vi "CreateNewWizard_Init.vi"(11 "Wizard":T1) -> (1 "Label":string, 2 "Enable Finish":bool, 3 "Enable Next":bool)   [LabVIEW 2020, in "Add Actor.lvlib"]
doc: "NI Confidential \n\n/**\n@brief This VI is called by the framework when an item of this type is first created.\n\n@author Joel Dixon\n\n@par Sample_Item_Init.vi\n This VI might typically set the popup menu for this item by calling mxLvSetPopupMenu.vi, set the icon for the item by calling mxLvSetIcon.vi, and set a name to be displayed in the tree by calling mxLvSetName.vi. \n\n@param \"Object\" [in] \nPassed by the framework as a reference to 'this' item in the tree. This parameter can be passed as the 'item' parameter for any of the mxLv** VIs, such as mxLvCreateItems.vi.\n*/"
uses:
  Add Actor.lvlib
  Support/Localized Strings.vi
  <resource>/Framework/Providers/API/ItemRef.ctl
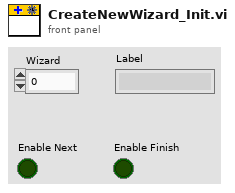
[diagram p1: front panel]
types:
  T1 = typedef "ItemRef.ctl" = u64
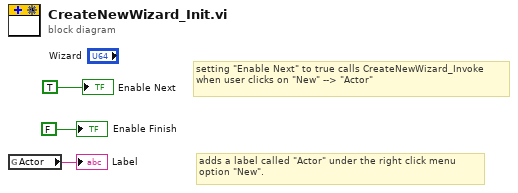
[diagram p0: block diagram]
diagram:
  # "adds a label called \"Actor\" under the right click menu \noption \"New\"."
  # "setting \"Enable Next\" to true calls CreateNewWizard_Invoke\nwhen user clicks on \"New\" --> \"Actor\""
  n1 = global read "Localized Strings.vi" "Actor"() -> (→"Label":string)
  "Enable Next" <- TRUE
  "Enable Finish" <- FALSE
